vi "Read Data and Draw to LV Picture_modif_RGB.vi"(6 "Pixel Format":string, 7 "Picture Ref":refnum<vi>, 8 "error in (no error)":errorcluster, 9 "Énum":enum16{"Grayscale", "Rainbow"}(ring), 10 "Data Cam Processing":T1, 11 "Buffer in":refnum<class "Buffer.lvclass">) -> (0 "error out":errorcluster, 2 "Picture":picture, 3 "Buffer out":refnum<class "Buffer.lvclass">, 5 "Data Cam Processing 2":T1)   [LabVIEW 2026]
uses:
  <vilib>/Serenial/G Industrial Camera/g_industrial_cam/Buffer/Buffer.lvclass
  Data-Processing.ctl
  <vilib>/picture/picture.llb/imagedata.ctl
  <vilib>/Serenial/G Industrial Camera/g_industrial_cam/Buffer/Buffer.lvclass/Buffer.ctl
  <vilib>/Serenial/G Industrial Camera/g_industrial_cam/Buffer/Draw Mono8 to Picture.vi
  <vilib>/Serenial/G Industrial Camera/g_industrial_cam/Buffer/Read as Pixmap Mono8.vi
  <vilib>/Serenial/G Industrial Camera/g_industrial_cam/Buffer/Draw Mono10 to Picture.vi
  <vilib>/Serenial/G Industrial Camera/g_industrial_cam/Buffer/Draw Mono12 to Picture.vi
  <vilib>/Serenial/G Industrial Camera/g_industrial_cam/Buffer/Draw Mono14 to Picture.vi
  <vilib>/Serenial/G Industrial Camera/g_industrial_cam/Buffer/Draw Mono16 to Picture.vi
  <vilib>/Serenial/G Industrial Camera/g_industrial_cam/Buffer/Draw Mono10p to Picture.vi
  <vilib>/Serenial/G Industrial Camera/g_industrial_cam/Buffer/Draw Mono12p to Picture.vi
  <vilib>/Serenial/G Industrial Camera/g_industrial_cam/Buffer/Draw Mono14p to Picture.vi
  <vilib>/Serenial/G Industrial Camera/g_industrial_cam/Buffer/Draw RGB8 to Picture.vi
  <vilib>/Serenial/G Industrial Camera/g_industrial_cam/Buffer/Draw BGR8 to Picture.vi
  <vilib>/Serenial/G Industrial Camera/g_industrial_cam/Buffer/DrawToPictureCore.vi
  <vilib>/Serenial/G Industrial Camera/g_industrial_cam/Buffer/ReadAsPixmapCore.vi
  <vilib>/Serenial/G Industrial Camera/g_industrial_cam/Buffer/GetBufferImageDimensions.vi
  <vilib>/Serenial/G Industrial Camera/g_industrial_cam/Buffer/Read Data as Mono8 Image.vi
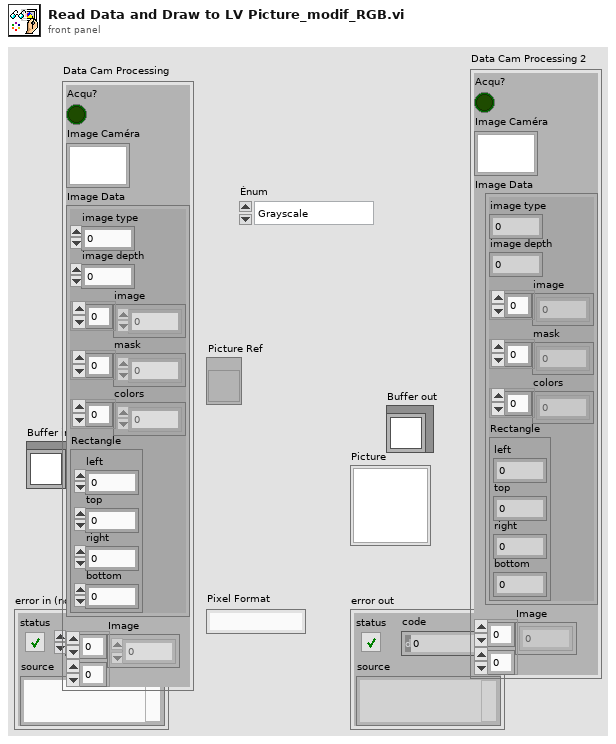
[diagram p1: front panel]
types:
  T1 = typedef "Data-Processing.ctl" = cluster{"Acqu?":bool, "Image Caméra":picture, "Image Data":T2, "Image":u8[][]}
  T2 = typedef "imagedata.ctl" = cluster{"image type":i32, "image depth":i32, "image":u8[], "mask":u8[], "colors":u32[], "Rectangle":cluster{"left":i16, "top":i16, "right":i16, "bottom":i16}}
  T3 = typedef "g_industrial_cam.lvlib/Buffer.lvclass/Image Size.ctl" = cluster{"Width":u16, "Height":u16}
  T4 = typedef "g_industrial_cam.lvlib/Buffer.lvclass/Picture Top Left Point Offset.ctl" = cluster{"x":i16, "y":i16}
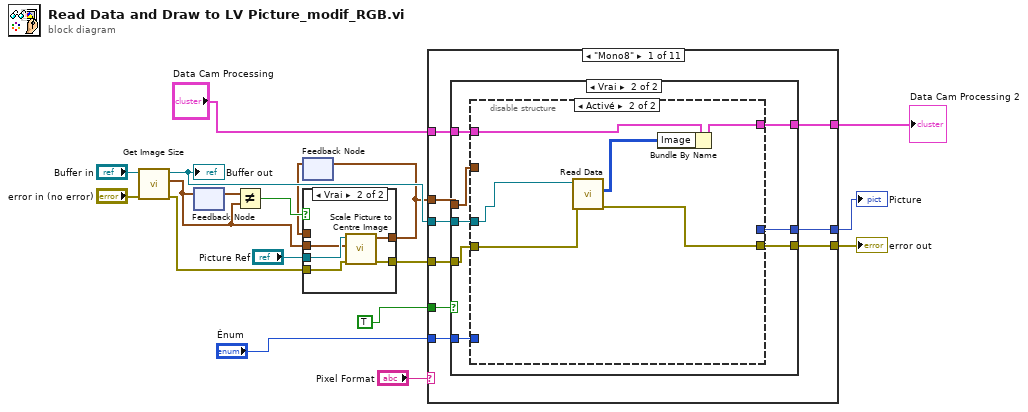
[diagram p0: block diagram]
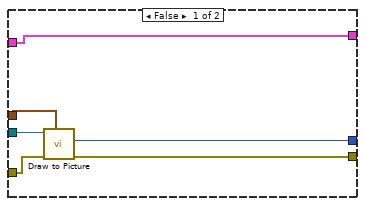
[diagram p3: hidden frame]
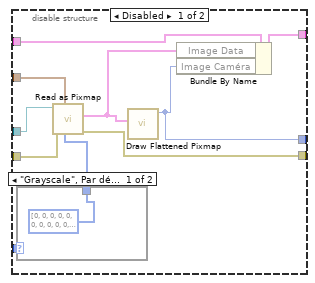
[diagram p4: hidden frame]
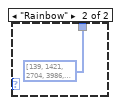
[diagram p5: hidden frame]
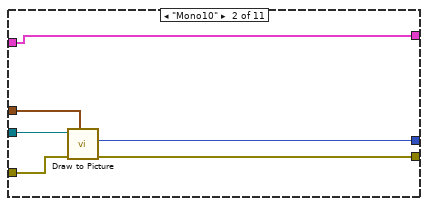
[diagram p6: hidden frame]
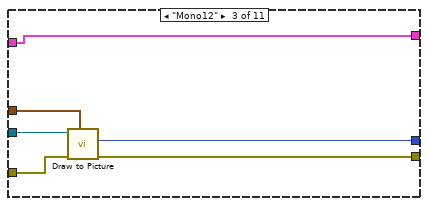
[diagram p7: hidden frame]
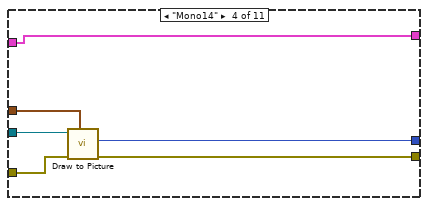
[diagram p8: hidden frame]
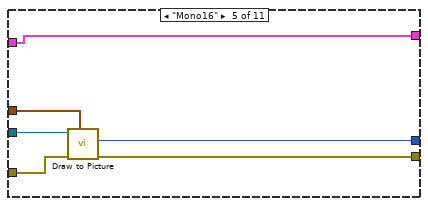
[diagram p9: hidden frame]
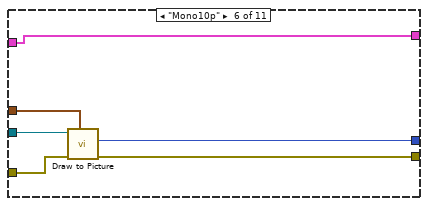
[diagram p10: hidden frame]
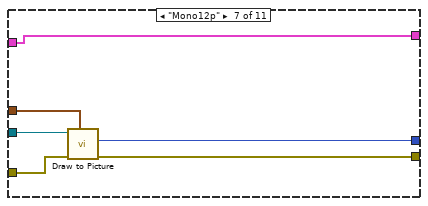
[diagram p11: hidden frame]
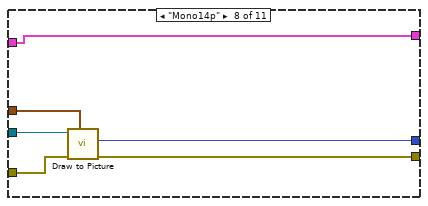
[diagram p12: hidden frame]
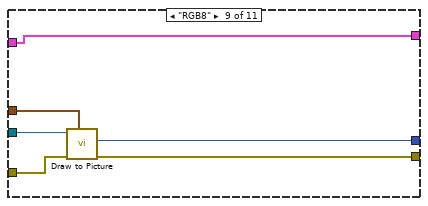
[diagram p13: hidden frame]
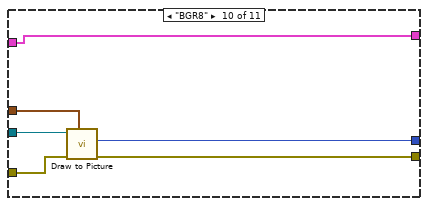
[diagram p14: hidden frame]
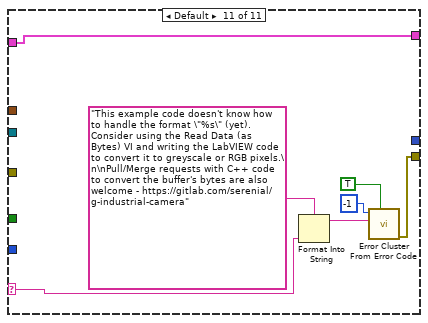
[diagram p15: hidden frame]
diagram:
  n1 = call <vilib>:"Get Image Size.vi"("error in (no error)"="error in (no error)", "Buffer in"="Buffer in") -> ("error out"=w11:errorcluster, "Image Size"=w8:T3, "Buffer"=w13:refnum<class "Buffer.lvclass">)  [unwired: 7 in]
  "Buffer out" <- w13
  n2 = feedback-in #1(w8) -> ()
  n3 = feedback #1() -> (w9:T3)  [unwired: 1 in]
  n4 = Not Equal?(x=w9, y=w8) -> (x != y?=w7:bool)
  n5 = feedback #2() -> (w5:T4)  [unwired: 1 in]
  n6 = case shown="Vrai" w7 {
    tunnel: "Picture Ref" -> [_ w25]
    tunnel: w11 -> [w20 w24]
    tunnel: [w19 w23] -> w6
    tunnel: [w20 w22] -> w10
    tunnel: w8 -> [_ w21]
    tunnel: w5 -> [w19 _]
    frame False {
    }
    frame True {
      n7 = call <vilib>:"Scale Picture to Centre Image.vi"("error in (no error)"=w24, "Image Size"=w21, "Picture in"=w25) -> ("error out"=w22:errorcluster, "Draw Image to Picture Offset"=w23:T4)  [unwired: 6 in, 1 out]
    }
  }
  n8 = feedback-in #2(w6) -> ()
  n9 = case shown="\"Mono8\"" "Pixel Format" {
    selector: "Pixel Format" -> [_ _ _ _ _ _ _ _ _ _ w122]
    tunnel: w13 -> [w34 w72 w78 w84 w90 w96 w102 w108 w114 w120 _]
    tunnel: [w33 w71 w77 w83 w89 w95 w101 w107 w113 w118 w123] -> w17
    tunnel: [w32 w70 w76 w82 w88 w94 w100 w106 w112 w119 _] -> w18
    tunnel: w6 -> [w31 w69 w75 w80 w86 w93 w99 w105 w111 w117 _]
    tunnel: w10 -> [w30 w68 w74 w81 w87 w92 w98 w104 w110 w116 _]
    tunnel: TRUE -> [w29 _ _ _ _ _ _ _ _ _ _]
    tunnel: [w28 w67 w73 w79 w85 w91 w97 w103 w109 w115 w121] -> w3
    tunnel: "Data Cam Processing" -> [w27 w67 w73 w79 w85 w91 w97 w103 w109 w115 w121]
    tunnel: "Énum" -> [w26 _ _ _ _ _ _ _ _ _ _]
    frame "Mono8" {
      n10 = case shown="Vrai" w29 {
        tunnel: w34 -> [w40 w46]
        tunnel: [w39 w45] -> w33
        tunnel: [w38 w42] -> w32
        tunnel: w31 -> [w37 w47]
        tunnel: w30 -> [w36 w48]
        tunnel: [w35 w43] -> w28
        tunnel: w27 -> [w35 w44]
        tunnel: w26 -> [_ w41]
        frame False {
          n11 = call-poly <vilib>:"Draw to Picture.vi"("Top Left Point (0,0)"=w37, "error in (no error)"=w36, "Buffer in"=w40) -> ("error out"=w39:errorcluster, "Picture"=w38:picture)  [unwired: 6 in, 1 out]
        }
        frame True {
          n12 = disable-structure shown="Activé" {
            disable-tunnel: w48 -> [w58 w64]
            disable-tunnel: w47 -> [w57 _]
            disable-tunnel: w46 -> [w56 w65]
            disable-tunnel: [w55 w63] -> w45
            disable-tunnel: w44 -> [w53 w66]
            disable-tunnel: [w52 w62] -> w43
            disable-tunnel: [w50 _] -> w42
            disable-tunnel: w41 -> [w49 _]
            frame Disabled {
              n13 = case shown="\"Grayscale\", Par défaut" w49 {
                tunnel: [u8[] [0, 0, 0, 0, 0, 0, 0, 0, 0, 0, 0, 0, 0, 0, 0, 0, 0, 0, 0, 0, 0, 0, 0, 0, 0, 0, 0, 0, 0, 0, 0, 0, 0, 0, 0, 0, 0, 0, 0, 0, 0, 0, 0, 0, 0, 0, 0, 0, 0, 0, 0, 0, 0, 0, 0, 0, 0, 0, 0, 0, 0, 0, 0, 0, 0, 0, 0, 0, 0, 0, 0, 0, 0, 0, 0, 0, 0, 0, 0, 0, 0, 0, 0, 0, 0, 0, 0, 0, 0, 0, 0, 0, 0, 0, 0, 0, 0, 0, 0, 0, 0, 0, 0, 0, 0, 0, 0, 0, 0, 0, 0, 0, 0, 0, 0, 0, 0, 0, 0, 0, 0, 0, 0, 0, 0, 0, 0, 0, 0, 0, 0, 0, 0, 0, 0, 0, 0, 0, 0, 0, 0, 0, 0, 0, 0, 0, 0, 0, 0, 0, 0, 0, 0, 0, 0, 0, 0, 0, 0, 0, 0, 0, 0, 0, 0, 0, 0, 0, 0, 0, 0, 0, 0, 0, 0, 0, 0, 0, 0, 0, 0, 0, 0, 0, 0, 0, 0, 0, 0, 0, 0, 0, 0, 0, 0, 0, 0, 0, 0, 0, 0, 0, 0, 0, 0, 0, 0, 0, 0, 0, 0, 0, 0, 0, 0, 0, 0, 0, 0, 0, 0, 0, 0, 0, 0, 0, 0, 0, 0, 0, 0, 0, 0, 0, 0, 0, 0, 0, 0, 0, 0, 0, 0, 0, 0, 0, 0, 0, 0, 0, 0, 0, 0, 0, 0, 0] ("Tableau 2") u32[] [139, 1421, 2704, 3986, 5268, 6550, 7833, 9115, 10397, 11679, 12962, 14244, 15526, 16809, 18091, 19373, 20655, 21938, 23220, 24502, 25784, 27067, 28349, 29631, 30914, 32196, 33478, 34760, 36043, 37325, 38607, 39890, 41172, 42454, 43736, 45019, 46301, 47583, 48865, 50148, 51430, 52712, 53995, 55277, 56559, 57841, 59124, 60406, 61688, 62970, 64253, 65535, 65530, 65525, 65520, 65515, 65510, 65505, 65500, 65495, 65490, 65485, 65480, 65475, 65470, 65465, 65460, 65455, 65450, 65445, 65440, 65435, 65430, 65425, 65420, 65415, 65410, 65405, 65400, 65395, 65390, 65385, 65380, 65375, 65370, 65365, 65360, 65355, 65350, 65345, 65340, 65335, 65330, 65325, 65320, 65315, 65310, 65305, 65300, 65295, 65290, 65285, 65280, 392960, 720640, 1048320, 1376000, 1703680, 2031360, 2359040, 2686720, 3014400, 3342080, 3669760, 3997440, 4325120, 4652800, 4980480, 5308160, 5635840, 5963520, 6291200, 6618880, 6946560, 7274240, 7601920, 7929600, 8257280, 8584960, 8912640, 9240320, 9568000, 9895680, 10223360, 10551040, 10878720, 11206400, 11534080, 11861760, 12189440, 12517120, 12844800, 13172480, 13500160, 13827840, 14155520, 14483200, 14810880, 15138560, 15466240, 15793920, 16121600, 16449280, 16776960, 16775680, 16774400, 16773120, 16771840, 16770560, 16769280, 16768000, 16766720, 16765440, 16764160, 16762880, 16761600, 16760320, 16759040, 16757760, 16756480, 16755200, 16753920, 16752640, 16751360, 16750080, 16748800, 16747520, 16746240, 16744960, 16743680, 16742400, 16741120, 16739840, 16738560, 16737280, 16736000, 16734720, 16733440, 16732160, 16730880, 16729600, 16728320, 16727040, 16725760, 16724480, 16723200, 16721920, 16720640, 16719360, 16718080, 16716800, 16715520, 16714240, 16712960, 16711680, 16712965, 16714250, 16715535, 16716820, 16718105, 16719390, 16720675, 16721960, 16723245, 16724530, 16725815, 16727100, 16728385, 16729670, 16730955, 16732240, 16733525, 16734810, 16736095, 16737380, 16738665, 16739950, 16741235, 16742520, 16743805, 16745090, 16746375, 16747660, 16748945, 16750230, 16751515, 16752800, 16754085, 16755370, 16756655, 16757940, 16759225, 16760510, 16761795, 16763080, 16764365, 16765650, 16766935, 16768220, 16769505, 16770790, 16772075, 16773360, 16774645, 16775930, 16777215] ("Tableau")] -> w54
                frame "Grayscale", Default {
                }
                frame "Rainbow" {
                }
              }
              n14 = call-poly <vilib>:"Read as Pixmap.vi"("Colours (Empty: Use Greyscale)"=w54, "Top Left Point (0,0)"=w57, "error in (no error)"=w58, "Buffer in"=w56) -> ("error out"=w55:errorcluster, "Image Data"=w51:T2)  [unwired: 5 in, 1 out]
              n15 = call <vilib>:"Draw Flattened Pixmap.vi"("image data"=w51) -> ("new picture"=w50:picture)  [unwired: 8 in]
              n16 = Bundle By Name(cluster=w53, "Image Data"=w51, "Image Caméra"=w50) -> (w52:T1)
            }
            frame Enabled {
              n17 = call-poly <vilib>:"Read Data.vi"("error in (no error)"=w64, "Buffer in"=w65) -> ("error out"=w63:errorcluster, "Image"=w61:u8[][])  [unwired: 7 in, 1 out]
              n18 = Bundle By Name(cluster=w66, "Image"=w61) -> (w62:T1)
            }
          }
        }
      }
    }
    frame "Mono10" {
      n19 = call-poly <vilib>:"Draw to Picture.vi"("Top Left Point (0,0)"=w69, "error in (no error)"=w68, "Buffer in"=w72) -> ("error out"=w71:errorcluster, "Picture"=w70:picture)  [unwired: 6 in, 1 out]
    }
    frame "Mono12" {
      n20 = call-poly <vilib>:"Draw to Picture.vi"("Top Left Point (0,0)"=w75, "error in (no error)"=w74, "Buffer in"=w78) -> ("error out"=w77:errorcluster, "Picture"=w76:picture)  [unwired: 6 in, 1 out]
    }
    frame "Mono14" {
      n21 = call-poly <vilib>:"Draw to Picture.vi"("Top Left Point (0,0)"=w80, "error in (no error)"=w81, "Buffer in"=w84) -> ("error out"=w83:errorcluster, "Picture"=w82:picture)  [unwired: 6 in, 1 out]
    }
    frame "Mono16" {
      n22 = call-poly <vilib>:"Draw to Picture.vi"("Top Left Point (0,0)"=w86, "error in (no error)"=w87, "Buffer in"=w90) -> ("error out"=w89:errorcluster, "Picture"=w88:picture)  [unwired: 6 in, 1 out]
    }
    frame "Mono10p" {
      n23 = call-poly <vilib>:"Draw to Picture.vi"("Top Left Point (0,0)"=w93, "error in (no error)"=w92, "Buffer in"=w96) -> ("error out"=w95:errorcluster, "Picture"=w94:picture)  [unwired: 6 in, 1 out]
    }
    frame "Mono12p" {
      n24 = call-poly <vilib>:"Draw to Picture.vi"("Top Left Point (0,0)"=w99, "error in (no error)"=w98, "Buffer in"=w102) -> ("error out"=w101:errorcluster, "Picture"=w100:picture)  [unwired: 6 in, 1 out]
    }
    frame "Mono14p" {
      n25 = call-poly <vilib>:"Draw to Picture.vi"("Top Left Point (0,0)"=w105, "error in (no error)"=w104, "Buffer in"=w108) -> ("error out"=w107:errorcluster, "Picture"=w106:picture)  [unwired: 6 in, 1 out]
    }
    frame "RGB8" {
      n26 = call-poly <vilib>:"Draw to Picture.vi"("Top Left Point (0,0)"=w111, "error in (no error)"=w110, "Buffer in"=w114) -> ("error out"=w113:errorcluster, "Picture"=w112:picture)  [unwired: 6 in, 1 out]
    }
    frame "BGR8" {
      n27 = call-poly <vilib>:"Draw to Picture.vi"("Top Left Point (0,0)"=w117, "error in (no error)"=w116, "Buffer in"=w120) -> ("error out"=w118:errorcluster, "Picture"=w119:picture)  [unwired: 6 in, 1 out]
    }
    frame Default {
      n28 = Format Into String(format string="This example code doesn't know how to handle the format \"%s\" (yet). Consider using the Read Data (as Bytes) VI and writing the LabVIEW code to convert it to greyscale or RGB pixels.\n\nPull/Merge requests with C++ code to convert the buffer's bytes are also welcome - https://gitlab.com/serenial/g-industrial-camera", w122) -> (resulting string=w127:string)  [unwired: 2 in, 1 out]
      n29 = call <vilib>:"Error Cluster From Error Code.vi"("show call chain? (False)"=TRUE, "error message (\"\")"=w127, "error code (0)"=-1) -> ("error out"=w123:errorcluster)  [unwired: 6 in]
    }
  }
  "error out" <- w17
  "Picture" <- w18
  "Data Cam Processing 2" <- w3
